vi "CLASE6.vi"() -> ()   [LabVIEW 2011]
panel:
  out "Aceptado":bool
  out "Edad":dbl
  in  "Experiencia":u16(ring) items=["Experiencia", "NO tiene experiecia"]
  in  "Tiene Titulo":u16(ring) items=["No tiene", "Tiene  titulo"]
  # "SE DEBE DE SELECCIONAR SI TIENE O NO TIENE TITULO, LUEGO\nSI TIENE EXPERIENCIA Y GENERAR LA EDAD ENTRE 20-70.\nES CONTRATADO SI LA EDAD ES MAYOR  25 Y SI TIENE EXPERIENCIA O SI TIENE TITULO Y NO TIENE EXPERIENCIA\nY ES MAOYR A 25"
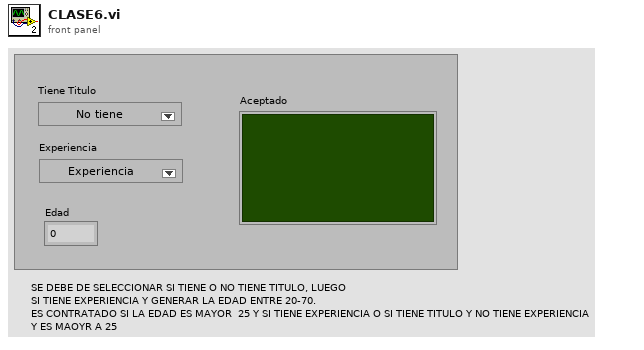
[diagram p1: front panel]
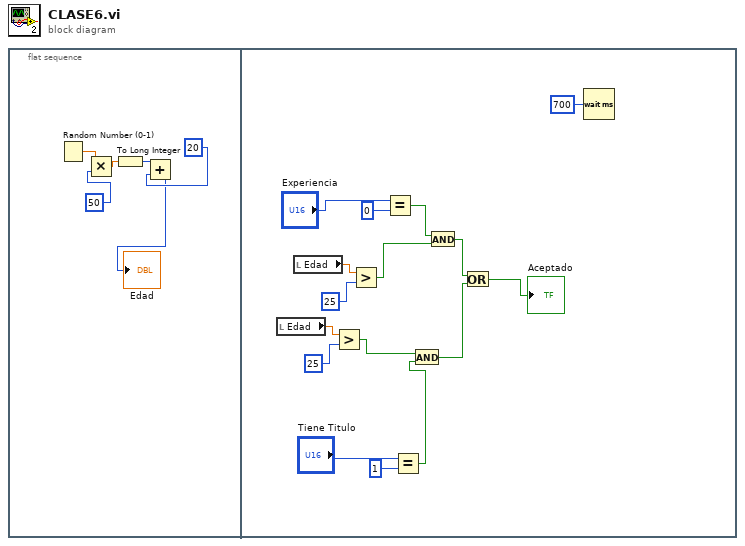
[diagram p0: block diagram]
diagram:
  n1 = flat-sequence {
    frame #0 {
      n2 = Random Number (0-1)() -> (number: 0 to 1=w5:dbl)
      n3 = Multiply(x=w5, y=50) -> (x*y=w4:dbl)
      n4 = To Long Integer(number=w4) -> (32bit integer=w3:i32)
      n5 = Add(x=w3, y=20) -> (x+y=→"Edad":i32)
    }
    frame #1 {
      n6 = local read "Edad"() -> (w16:dbl)
      n7 = local read "Edad"() -> (w21:dbl)
      n8 = Greater?(x=w16, y=25) -> (0:w12:bool)
      n9 = Greater?(x=w21, y=25) -> (0:w18:bool)
      n10 = Equal?(x="Experiencia", y=u16 0) -> (x = y?=w17:bool)
      n11 = Equal?(x="Tiene Titulo", y=u16 1) -> (x = y?=w11:bool)
      n12 = And(x=w12, y=w11) -> (x .and. y?=w9:bool)
      n13 = And(x=w17, y=w18) -> (x .and. y?=w10:bool)
      n14 = Or(x=w10, y=w9) -> (x .or. y?=→"Aceptado":bool)
      n15 = Wait (ms)(milliseconds to wait=u32 700) -> ()  [unwired: 1 out]
    }
  }
